vi "calc_CRC.vi"(1 "data":u8, 2 "address":u8, 3 "command":u8) -> (0 "CRC":u8)   [LabVIEW 2018]
doc: "calculates the CRC by XOR'ing the 3 bytes"
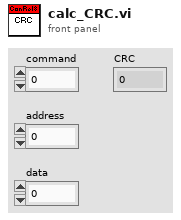
[diagram p1: front panel]
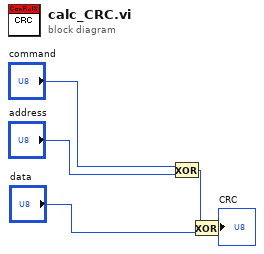
[diagram p0: block diagram]
diagram:
  n1 = Exclusive Or(1:"address", 2:"command") -> (0:w2:u8)
  n2 = Exclusive Or(1:"data", 2:w2) -> (0:→"CRC":u8)
